vi "UID Does Not Exist--error.vi"() -> (2 "Error":errorcluster)   [LabVIEW 2020, in "jettl.lvlib"]
uses:
  jettl.lvlib
  <vilib>/AdvancedString/Delimited String to 1D String Array.vi
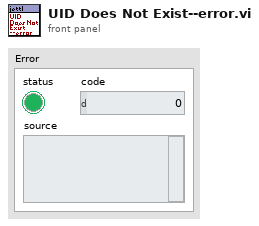
[diagram p1: front panel]
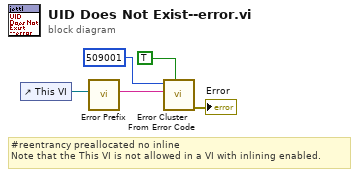
[diagram p0: block diagram]
diagram:
  # "#reentrancy preallocated no inline\nNote that the This VI is not allowed in a VI with inlining enabled."
  n1 = control-ref of="This VI"() -> (w4:refnum<vi>)
  n2 = call "Error Prefix.vi"("VI Ref"=w4) -> ("Prefix"=w3:string)  [unwired: 10 in]
  n3 = call <vilib>:"Error Cluster From Error Code.vi"("show call chain? (False)"=TRUE, "error message (\"\")"=w3, "error code (0)"=509001) -> ("error out"=→"Error":errorcluster)  [unwired: 6 in]
